vi "Apply Solver.vi"(6 "wait for reply (T)":bool=TRUE, 8 "error in":errorcluster, 9 "Number of Runs (1)":i32=1, 10 "Solver VI":path) -> (0 "error out":errorcluster, 1 "timed out?":bool, 2 "Detailed Results":string, 3 "Average Solve Count":dbl)   [LabVIEW 2020, in "Wordle Engine.lvlib"]
doc: "Applies a Solver VI to a specified number of Wordle words.\n_____\nCreated using DQMH Event Scripter 6.1.0.127."
uses:
  Wordle Engine.lvlib
  Apply Solver Argument--cluster.ctl
  Apply Solver (Reply Payload)--cluster.ctl
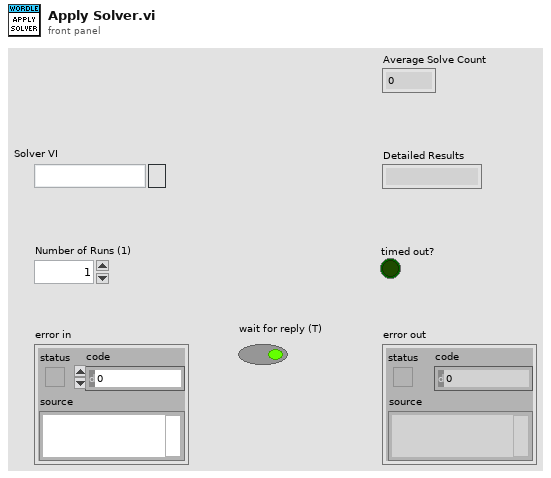
[diagram p1: front panel]
types:
  T1 = typedef "Wordle Engine.lvlib/Request Events--cluster.ctl" = cluster{"Stop Module":refnum<user-event>, "Show Panel":refnum<user-event>, "Hide Panel":refnum<user-event>, "Get Module Execution Status":refnum<user-event>, "Show Diagram":refnum<user-event>, "Select New Word":refnum<user-event>, "Make a Guess":refnum<user-event>, "Apply Solver":refnum<user-event>}
  T2 = typedef "Wordle Engine.lvlib/Apply Solver Argument--cluster.ctl" = cluster{"Solver VI":path, "Number of Runs (1)":i32, "Wait Notifier":refnum<notifier>, "wait for reply":bool}
  T3 = typedef "Wordle Engine.lvlib/Apply Solver (Reply Payload)--cluster.ctl" = cluster{"Average Solve Count":dbl, "Detailed Results":string, "error":errorcluster}
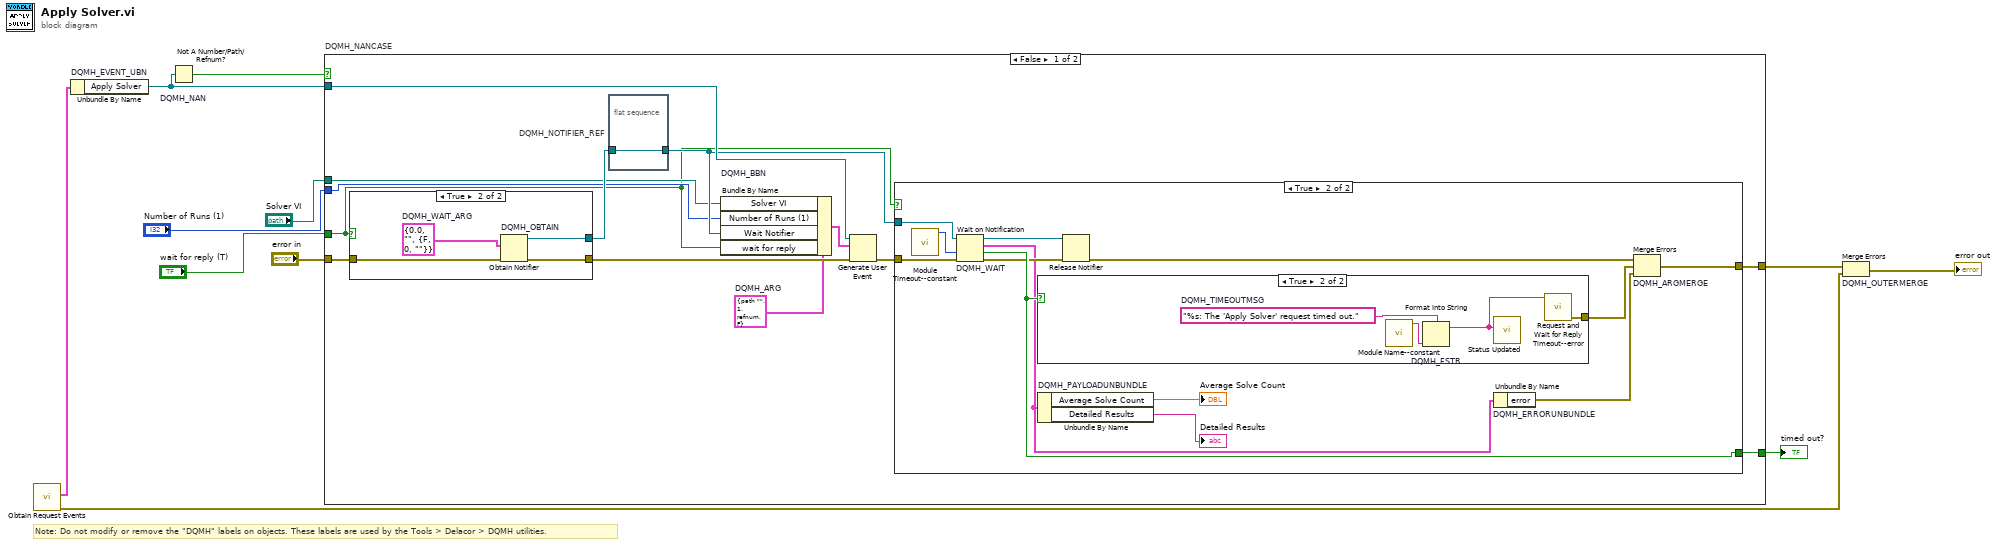
[diagram p0: block diagram]
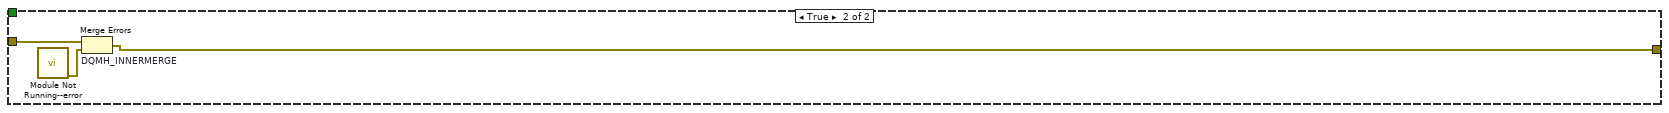
[diagram p5: hidden frame]
diagram:
  # "Note: Do not modify or remove the \"DQMH\" labels on objects. These labels are used by the Tools > Delacor > DQMH utilities."
  n1 = call "Obtain Request Events.vi"() -> ("error out"=w2:errorcluster, "Wordle Engine Request Events"=w1:T1)  [unwired: 10 in]
  n2 = Unbundle By Name "DQMH_EVENT_UBN"(w1) -> ("Apply Solver"=w9:refnum<user-event>)
  n3 = Not A Number/Path/Refnum? "DQMH_NAN"(number/path/refnum=w9) -> (NaN/Path/Refnum?=w8:bool)
  n4 = case "DQMH_NANCASE" shown="False" w8 {
    tunnel: "error in" -> [w24 w51]
    tunnel: w9 -> [w22 _]
    tunnel: [w19 w50] -> w6
    tunnel: [w20 _] -> w7
    tunnel: "Solver VI" -> [w15 _]
    tunnel: "Number of Runs (1)" -> [w14 _]
    tunnel: "wait for reply (T)" -> [w13 _]
    frame False {
      w12 = T2 {"Solver VI"=path "", "Number of Runs (1)"=1, "Wait Notifier"=refnum, "wait for reply"=FALSE}  # DQMH_ARG
      n5 = case shown="True" w13 {
        tunnel: w24 -> [w44 w48]
        tunnel: [w44 w47] -> w21
        tunnel: [_ w45] -> w17
        frame False {
        }
        frame True {
          w46 = T3 {"Average Solve Count"=0.0, "Detailed Results"="", "error"={"status"=FALSE, "code"=0, "source"=""}}  # DQMH_WAIT_ARG
          n6 = Obtain Notifier "DQMH_OBTAIN"(notification data type=w46, error in (no error)=w48) -> (notifier out=w45:refnum<notifier>, error out=w47:errorcluster)  [unwired: 2 in, 1 out]
        }
      }
      n7 = flat-sequence "DQMH_NOTIFIER_REF" {
        tunnel: w17 -> [w25]
        tunnel: [w25] -> w16
        frame #0 {
        }
      }
      n8 = Bundle By Name "DQMH_BBN"(cluster=w12, "Solver VI"=w15, "Number of Runs (1)"=w14, "Wait Notifier"=w16, "wait for reply"=w13) -> (w18:T2)
      n9 = Generate User Event(user event=w22, event data cluster=w18, error in=w21) -> (error out=w23:errorcluster)  [unwired: 1 in, 1 out]
      n10 = case shown="True" w13 {
        tunnel: w23 -> [w26 w39]
        tunnel: w16 -> [_ w38]
        tunnel: [_ w36] -> w20
        tunnel: [w26 w35] -> w19
        frame False {
        }
        frame True {
          n11 = call "Module Timeout--constant.vi"() -> ("Module Timeout"=w29:i32)  [unwired: 11 in]
          n12 = Wait on Notification "DQMH_WAIT"(notifier=w38, timeout in ms (-1)=w29, error in (no error)=w39) -> (notifier out=w37:refnum<notifier>, notification=w30:T3, timed out?=w36:bool, error out=w34:errorcluster)  [unwired: 1 in]
          n13 = case shown="True" w36 {
            tunnel: [_ w41] -> w31
            frame False {
            }
            frame True {
              w43 = "%s: The 'Apply Solver' request timed out."  # DQMH_TIMEOUTMSG
              n14 = call "Module Name--constant.vi"() -> ("Module Name"=w40:string)  [unwired: 11 in]
              n15 = Format Into String "DQMH_FSTR"(format string=w43, w40) -> (resulting string=w42:string)  [unwired: 2 in, 1 out]
              n16 = call "Status Updated.vi"("Status"=w42) -> ()  [unwired: 10 in, 1 out]
              n17 = call "Request and Wait for Reply Timeout--error.vi"("Error Message"=w42) -> ("error out"=w41:errorcluster)  [unwired: 10 in]
            }
          }
          n18 = Unbundle By Name "DQMH_PAYLOADUNBUNDLE"(w30) -> ("Average Solve Count"=→"Average Solve Count":dbl, "Detailed Results"=→"Detailed Results":string)
          n19 = Release Notifier(notifier=w37, error in (no error)=w34) -> (error out=w33:errorcluster)  [unwired: 1 in, 2 out]
          n20 = Unbundle By Name "DQMH_ERRORUNBUNDLE"(w30) -> ("error"=w32:errorcluster)
          n21 = Merge Errors "DQMH_ARGMERGE"(w33, w31, w32) -> (w35:errorcluster)
        }
      }
    }
    frame True {
      n22 = call "Module Not Running--error.vi"() -> ("error out"=w49:errorcluster)  [unwired: 11 in]
      n23 = Merge Errors "DQMH_INNERMERGE"(w51, w49) -> (w50:errorcluster)
    }
  }
  "timed out?" <- w7
  n24 = Merge Errors "DQMH_OUTERMERGE"(w6, w2) -> (→"error out":errorcluster)
